vi "UTILITY General GEA Setup.vi"(8 "Error In":errorcluster, 10 "all rows In":string[][](array[string])) -> (0 "Error Out":errorcluster, 1 "Board Index":i32, 2 "all rows Out":string[][](array[string]), 3 "Board ID":string)   [LabVIEW 2020]
uses:
  <vilib>/Utility/error.llb/whitespace.ctl
  Drivers/GEA3 Toolkit/LabVIEW GEA3 Rev2 API Toolkit LV2016/library/GEA2_Toolkit.lvlib
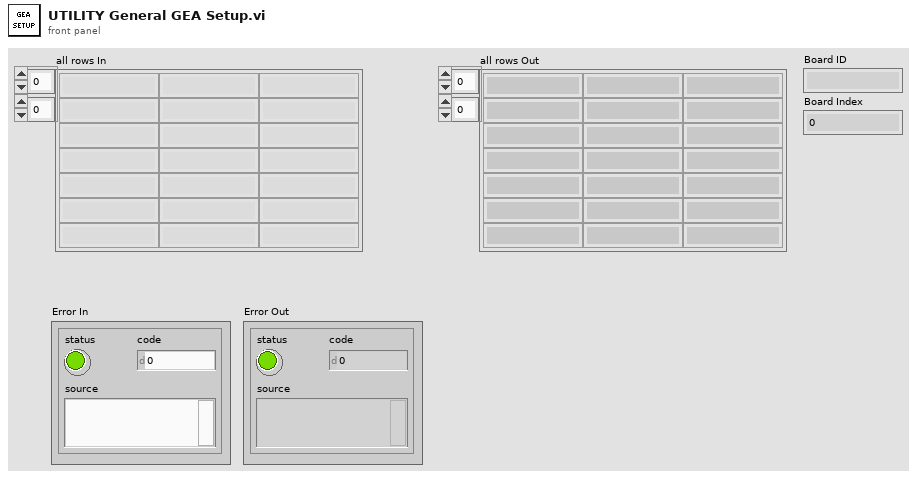
[diagram p1: front panel]
types:
  T1 = typedef "whitespace.ctl" = u16
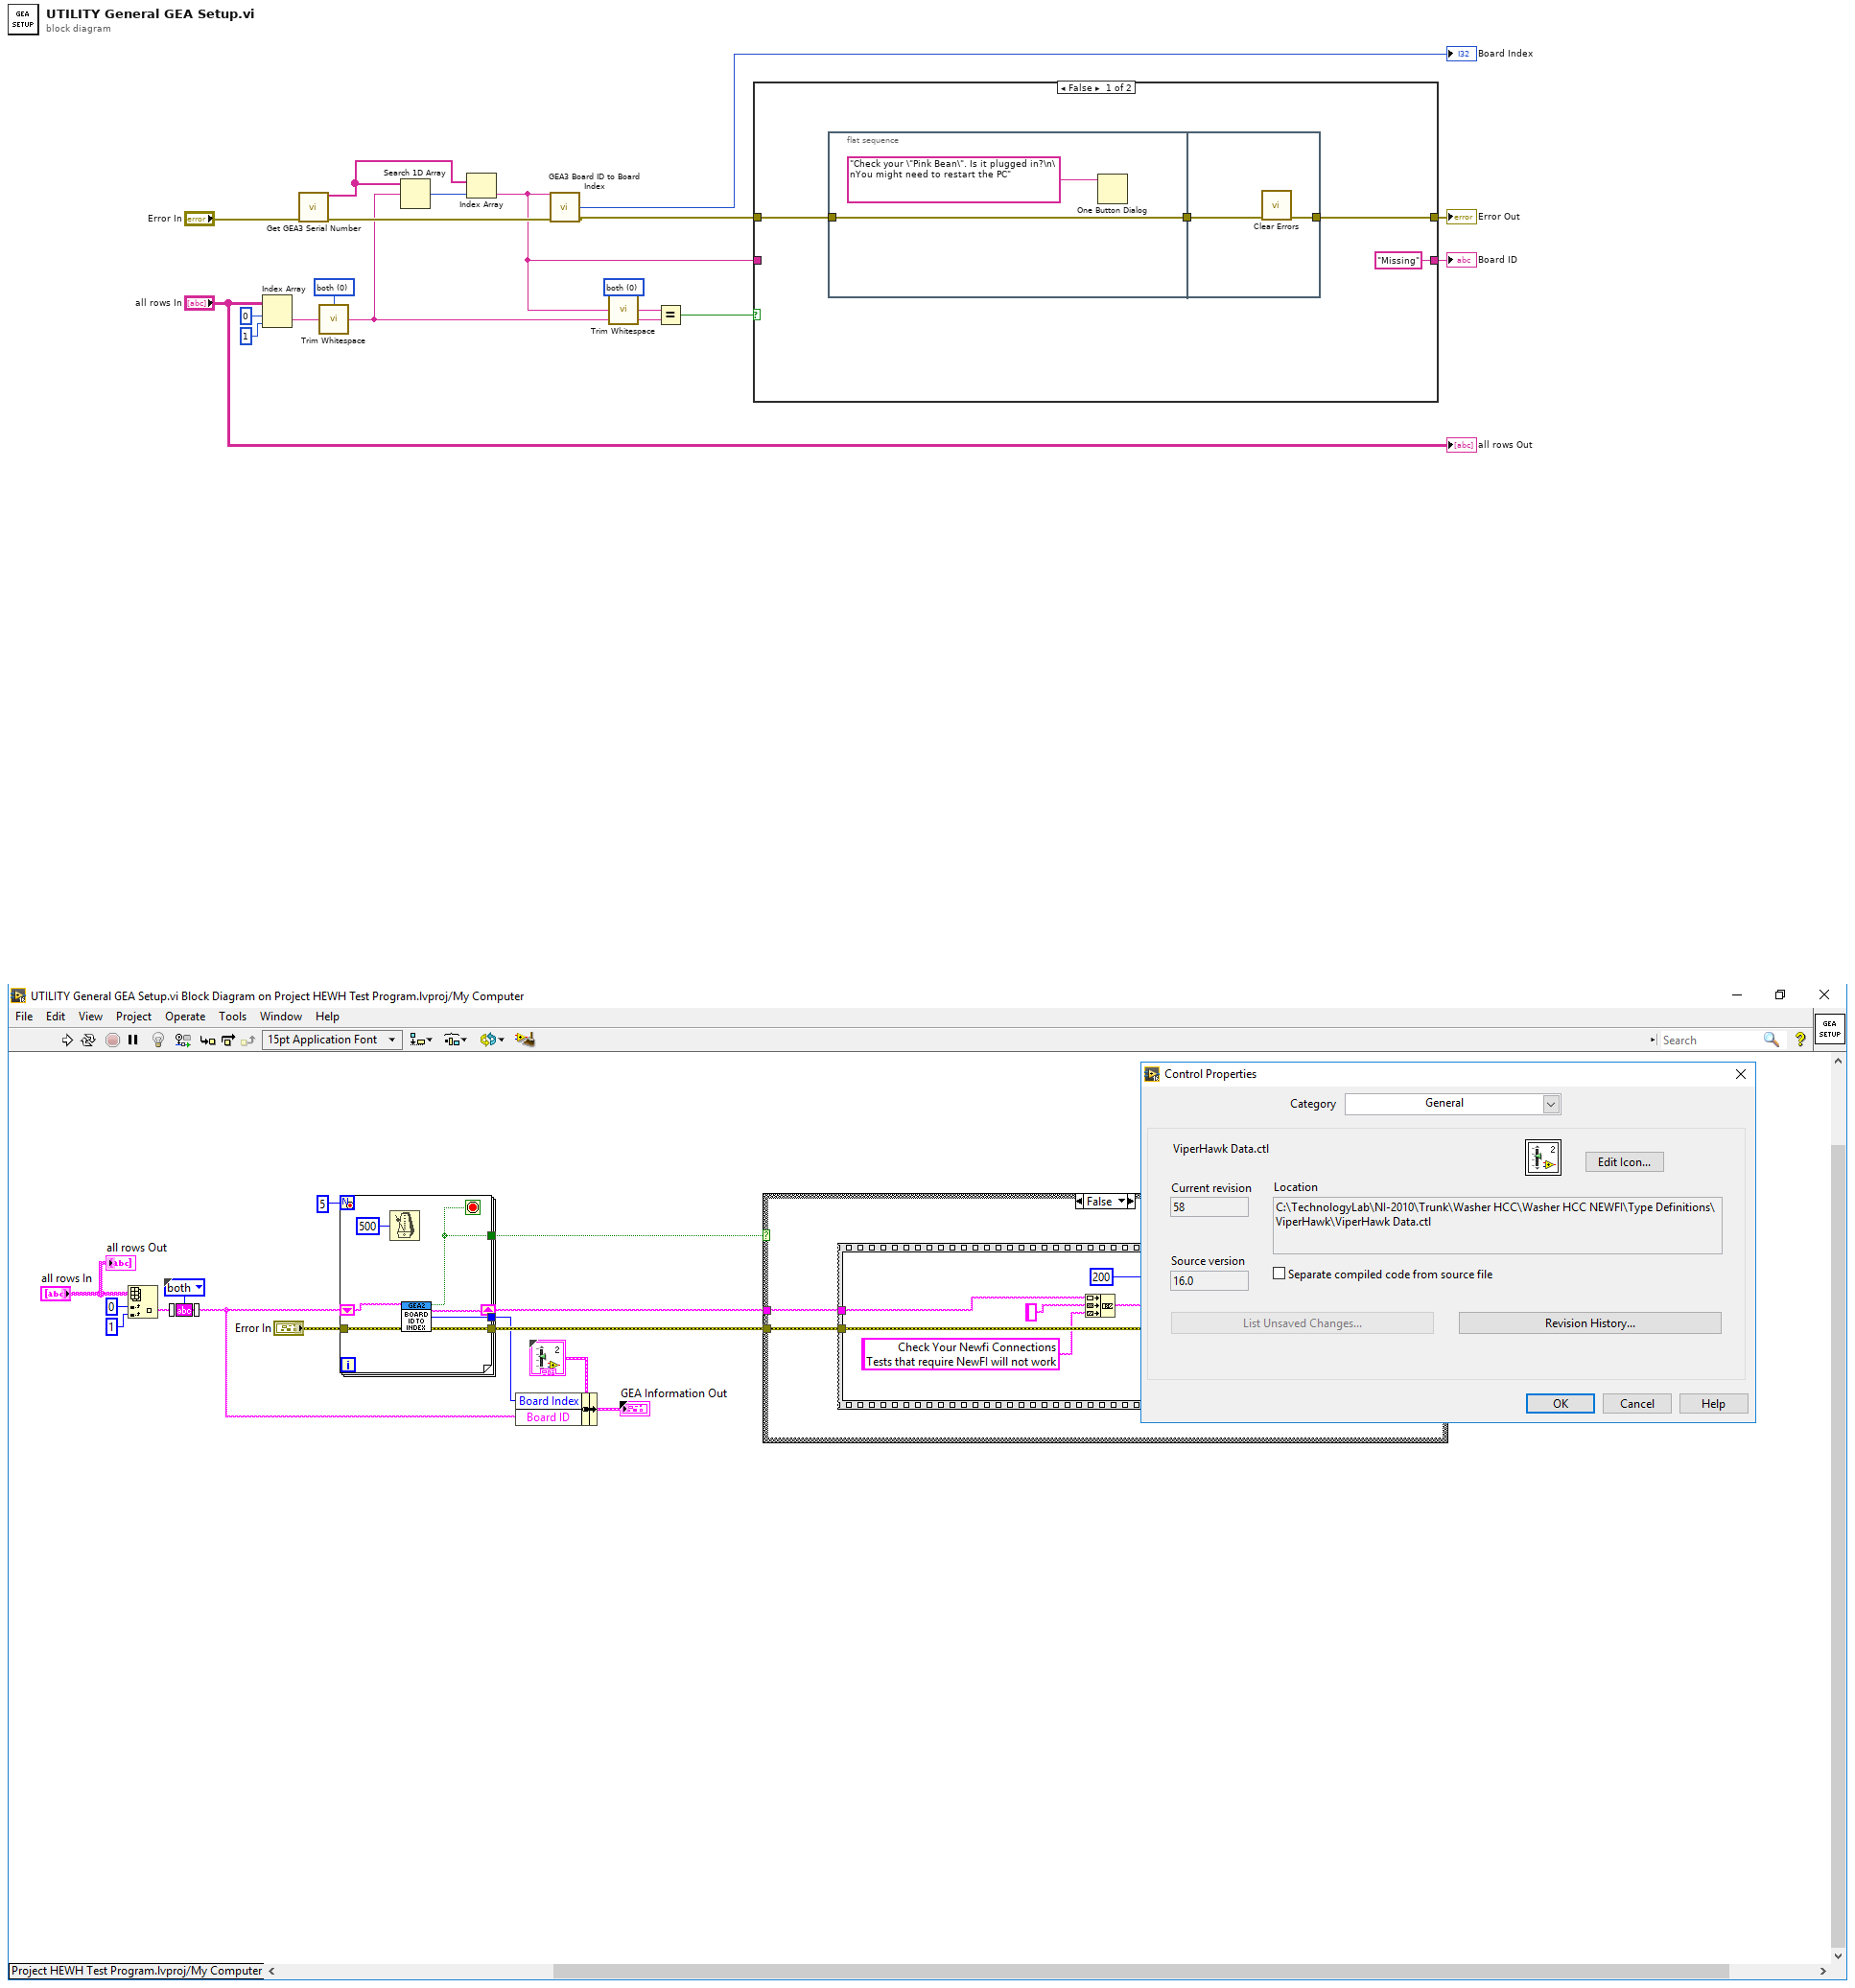
[diagram p0: block diagram]
diagram:
  w8 = T1 0 items=["both", "start of string", "end of string"] ("location (both)")
  w10 = T1 0 items=["both", "start of string", "end of string"] ("location (both)")
  n1 = Index Array(array="all rows In", index (row)=0 ("disabled index (row)"), index (col)=1 ("disabled index (col)")) -> (element=w17:string)
  n2 = call "Get GEA3 Serial Number.vi"("Error In"="Error In") -> ("GEA3 Serial Numbers"=w4:string[], "Error Out"=w9:errorcluster)  [unwired: 13 in]
  n3 = call <vilib>:"Trim Whitespace.vi"("string"=w17, "location (both)"=w10) -> ("trimmed string"=w5:string)
  n4 = Search 1D Array(1D array=w4, element=w5) -> (index of element=w3:i32)  [unwired: 1 in]
  n5 = Index Array(array=w4, index=w3) -> (element=w2:string)
  n6 = call "GEA3 Board ID to Board Index.vi"("GEA3 Serial Number"=w2, "Error In"=w9) -> ("Board Index"=→"Board Index":i32, "Error Out"=w12:errorcluster)  [unwired: 9 in, 3 out]
  n7 = call <vilib>:"Trim Whitespace.vi"("string"=w2, "location (both)"=w8) -> ("trimmed string"=w7:string)
  n8 = Equal?(x=w7, y=w5) -> (x = y?=w1:bool)
  n9 = case shown="False" w1 {
    tunnel: w12 -> [w22 w28]
    tunnel: [w21 w28] -> w11
    tunnel: w2 -> [_ w27]
    tunnel: ["Missing" ("Serial Number") w27] -> w6
    frame False {
      n10 = flat-sequence {
        tunnel: w22 -> [w24]
        tunnel: [w24] -> w20
        tunnel: [w25] -> w21
        tunnel: w20 -> [w26]
        frame #0 {
          n11 = One Button Dialog(message="Check your \"Pink Bean\". Is it plugged in?\n\nYou might need to restart the PC" ("string")) -> ()  [unwired: 1 in, 1 out]
        }
        frame #1 {
          n12 = call <vilib>:"Clear Errors.vi"("error in (no error)"=w26) -> ("error out"=w25:errorcluster)  [unwired: 5 in, 1 out]
        }
      }
    }
    frame True {
    }
  }
  "Error Out" <- w11
  "Board ID" <- w6
  "all rows Out" <- "all rows In"
